vi "FXP_state_space_feedforward_XY.vi"(5 "Ns_yff":u8=9, 6 "enable_FF":bool, 7 "Ns_xff":u8=9, 11 "Refxy":fxp<+/-,36,13>[](array[numeric])=[0.0, 0.0]) -> (3 "Refxy_ff":fxp<+/-,36,13>[](array[numeric]))   [LabVIEW 2017]
uses:
  fixed-point-ss/typeDefs/x_vec_bram.ctl
  fixed-point-ss/typeDefs/A_as_vec_bram.ctl
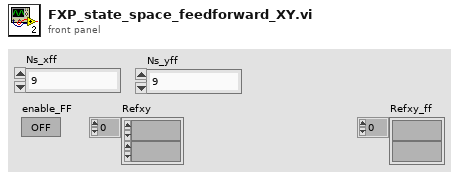
[diagram p1: front panel]
types:
  T1 = typedef "A_as_vec_bram.ctl" = refnum<k21>
  T2 = typedef "x_vec_bram.ctl" = refnum<k21>
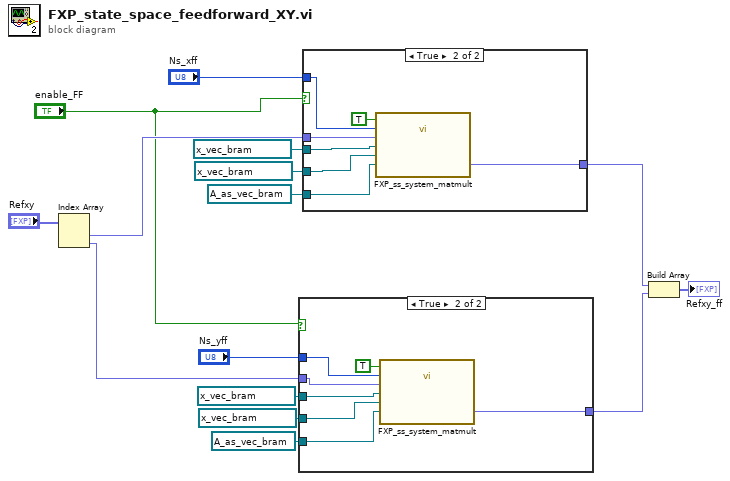
[diagram p0: block diagram]
diagram:
  n1 = Index Array(array="Refxy") -> (element #1=w4:fxp<+/-,36,13>, element #2=w5:fxp<+/-,36,13>)  [unwired: 2 in]
  n2 = case shown="True" "enable_FF" {
    tunnel: T1 "ABCD_yff" ("ABCD_as_col") -> [_ w23]
    tunnel: T2 "xk_1_0_yFF" ("Memory") -> [_ w21]
    tunnel: T2 "xk_0_1_yFF" ("Memory") -> [_ w20]
    tunnel: [w16 w19] -> w8
    tunnel: w5 -> [w16 w18]
    tunnel: "Ns_yff" -> [_ w17]
    frame False {
    }
    frame True {
      n3 = call "FXP_ss_system_matmult.vi"("xk_0_1"=w20, "xk_1_0"=w21, "ABCD_as_col"=w23, "Uk"=w18, "Ns_nsw"=w17, "inputValid"=TRUE) -> ("Yk"=w19:fxp<+/-,36,13>)  [unwired: 4 in, 1 out]
    }
  }
  n4 = case shown="True" "enable_FF" {
    tunnel: T1 "ABCD_xff" ("ABCD_as_col") -> [_ w31]
    tunnel: T2 "xk_1_0_xFF" ("Memory") -> [_ w29]
    tunnel: T2 "xk_0_1_xFF" ("Memory") -> [_ w28]
    tunnel: [w24 w27] -> w9
    tunnel: w4 -> [w24 w26]
    tunnel: "Ns_xff" -> [_ w25]
    frame False {
    }
    frame True {
      n5 = call "FXP_ss_system_matmult.vi"("xk_0_1"=w28, "xk_1_0"=w29, "ABCD_as_col"=w31, "Uk"=w26, "Ns_nsw"=w25, "inputValid"=TRUE) -> ("Yk"=w27:fxp<+/-,36,13>)  [unwired: 4 in, 1 out]
    }
  }
  n6 = Build Array(w9, w8) -> (→"Refxy_ff":fxp<+/-,36,13>[])
